vi "TimeOut.vi"(9 "IA State":T2={"our_robots"=[], "enemy_robots"=[], "balls"=[], "geometry"={"field_length"=0, "field_width"=0, "goal_width"=0, "goal_depth"=0, "center_circle_radius"=0, "defense_width"=0, "defense_depth"=0, "free_kick_from_defense_dist"=0, "penalty_spot_from_field_line_dist"=0, "penalty_line_from_spot_dist"=0, "half_moon_depth"=0, "half_moon_width"=0}, "IA Judge"={"stage"="", "command"="", "our_goalie_id"=0.0, "enemy_goalie_id"=0.0, "command enum"=enum."Halt", "Time"=enum."Azul"}, "Received Timestamp"=timestamp(0 s since 1904-01-01), "Events"={"Touch"=FALSE, "id touch"=0.0, "Ball out of \nVision"=FALSE, "Ball inside \nGoalie area"=FALSE, "Robot not responding"=FALSE, "Robots responding status"=[1.0, 1.0, 1.0, 1.0, 1.0, 1.0], "Enemy Ball \nPossession"=FALSE, "Id ini Possession"=0.0, "Ball Possesion"=FALSE, "Id Possesion"=0.0, "Ball at\nour goal side"=FALSE, "Ball at\ntouchline"=FALSE, "Ball at\nenemy goal side"=FALSE}}, 10 "balls":T1[](array[typedef]), 11 "Robot in":T3) -> (3 "Robot out":T3)   [LabVIEW 2018]
uses:
  AI Parameters.ctl
  Core/AI Robot.ctl
  Functions Enum.ctl
  AttackerStates.ctl
  Path Planning/RRT/PathDests.ctl
  Path Planning/RRT/PathDest.ctl
  Core/AI Input.ctl
  Core/AI Ball.ctl
  Core/Field Size.ctl
  Core/AI Judge.ctl
  Command Enum.ctl
  Util/Events/Events.ctl
panel:
  in  "AI Parameters":T12={"GotoKick"={"Dist do cone a frente"=0.0, "attacker farback"=1000.0, "Perto"=300.0, "min dist to kick"=0.0, "kick eps"=110.0, "Time to transition"=0.05}, "Attacker"={"CC chute"=0.09, "CC passe"=0.045, "Kick Force"=200.0, "D ball-robot Kick"=200.0, "D ball-robot Pass"=0.0}, "Defender"={"D max"=1700.0, "Vel p/ robô av"=1000.0, "Kick Force"=100.0, "D atk-def"=300.0, "D farback"=400.0}, "Timeout"={"Field/v in x"=6.0, "Dist Robots"=300, "Dist up in y"=300}, "Pose Striker"={"dist"=200.0, "Numeric"=-4.0, "dist 2"=200.0}, "Dist Stop"=300.0, "Distance when ball out"=200, "D central gap "=150.0, "T pass"=0.0, "Force ++"=0.0, "range kick"=0.0, "Chute alto"=TRUE, "Marcador novo"=TRUE} {"D central gap" format="%#_13g"; "Dist Stop" format="%#_13g"; "Pose Striker"."Numeric" format="%#_13g"; "Defender"."Kick Force" format="%#_13g"; "Defender"."Vel p/ robô av" format="%#_13g"; "Attacker"."D ball-robot Kick" format="%#_13g"; "Attacker"."Kick Force" format="%#_13g"; "Attacker"."CC passe" format="%#_13g"; "Attacker"."CC chute" format="%#_13g"; "GotoKick"."min dist to kick" format="%#_13g"; "GotoKick"."Perto" format="%#_13g"; "GotoKick"."attacker farback" format="%#_13g"; "GotoKick"."Dist do cone a frente" format="%#_13g"}
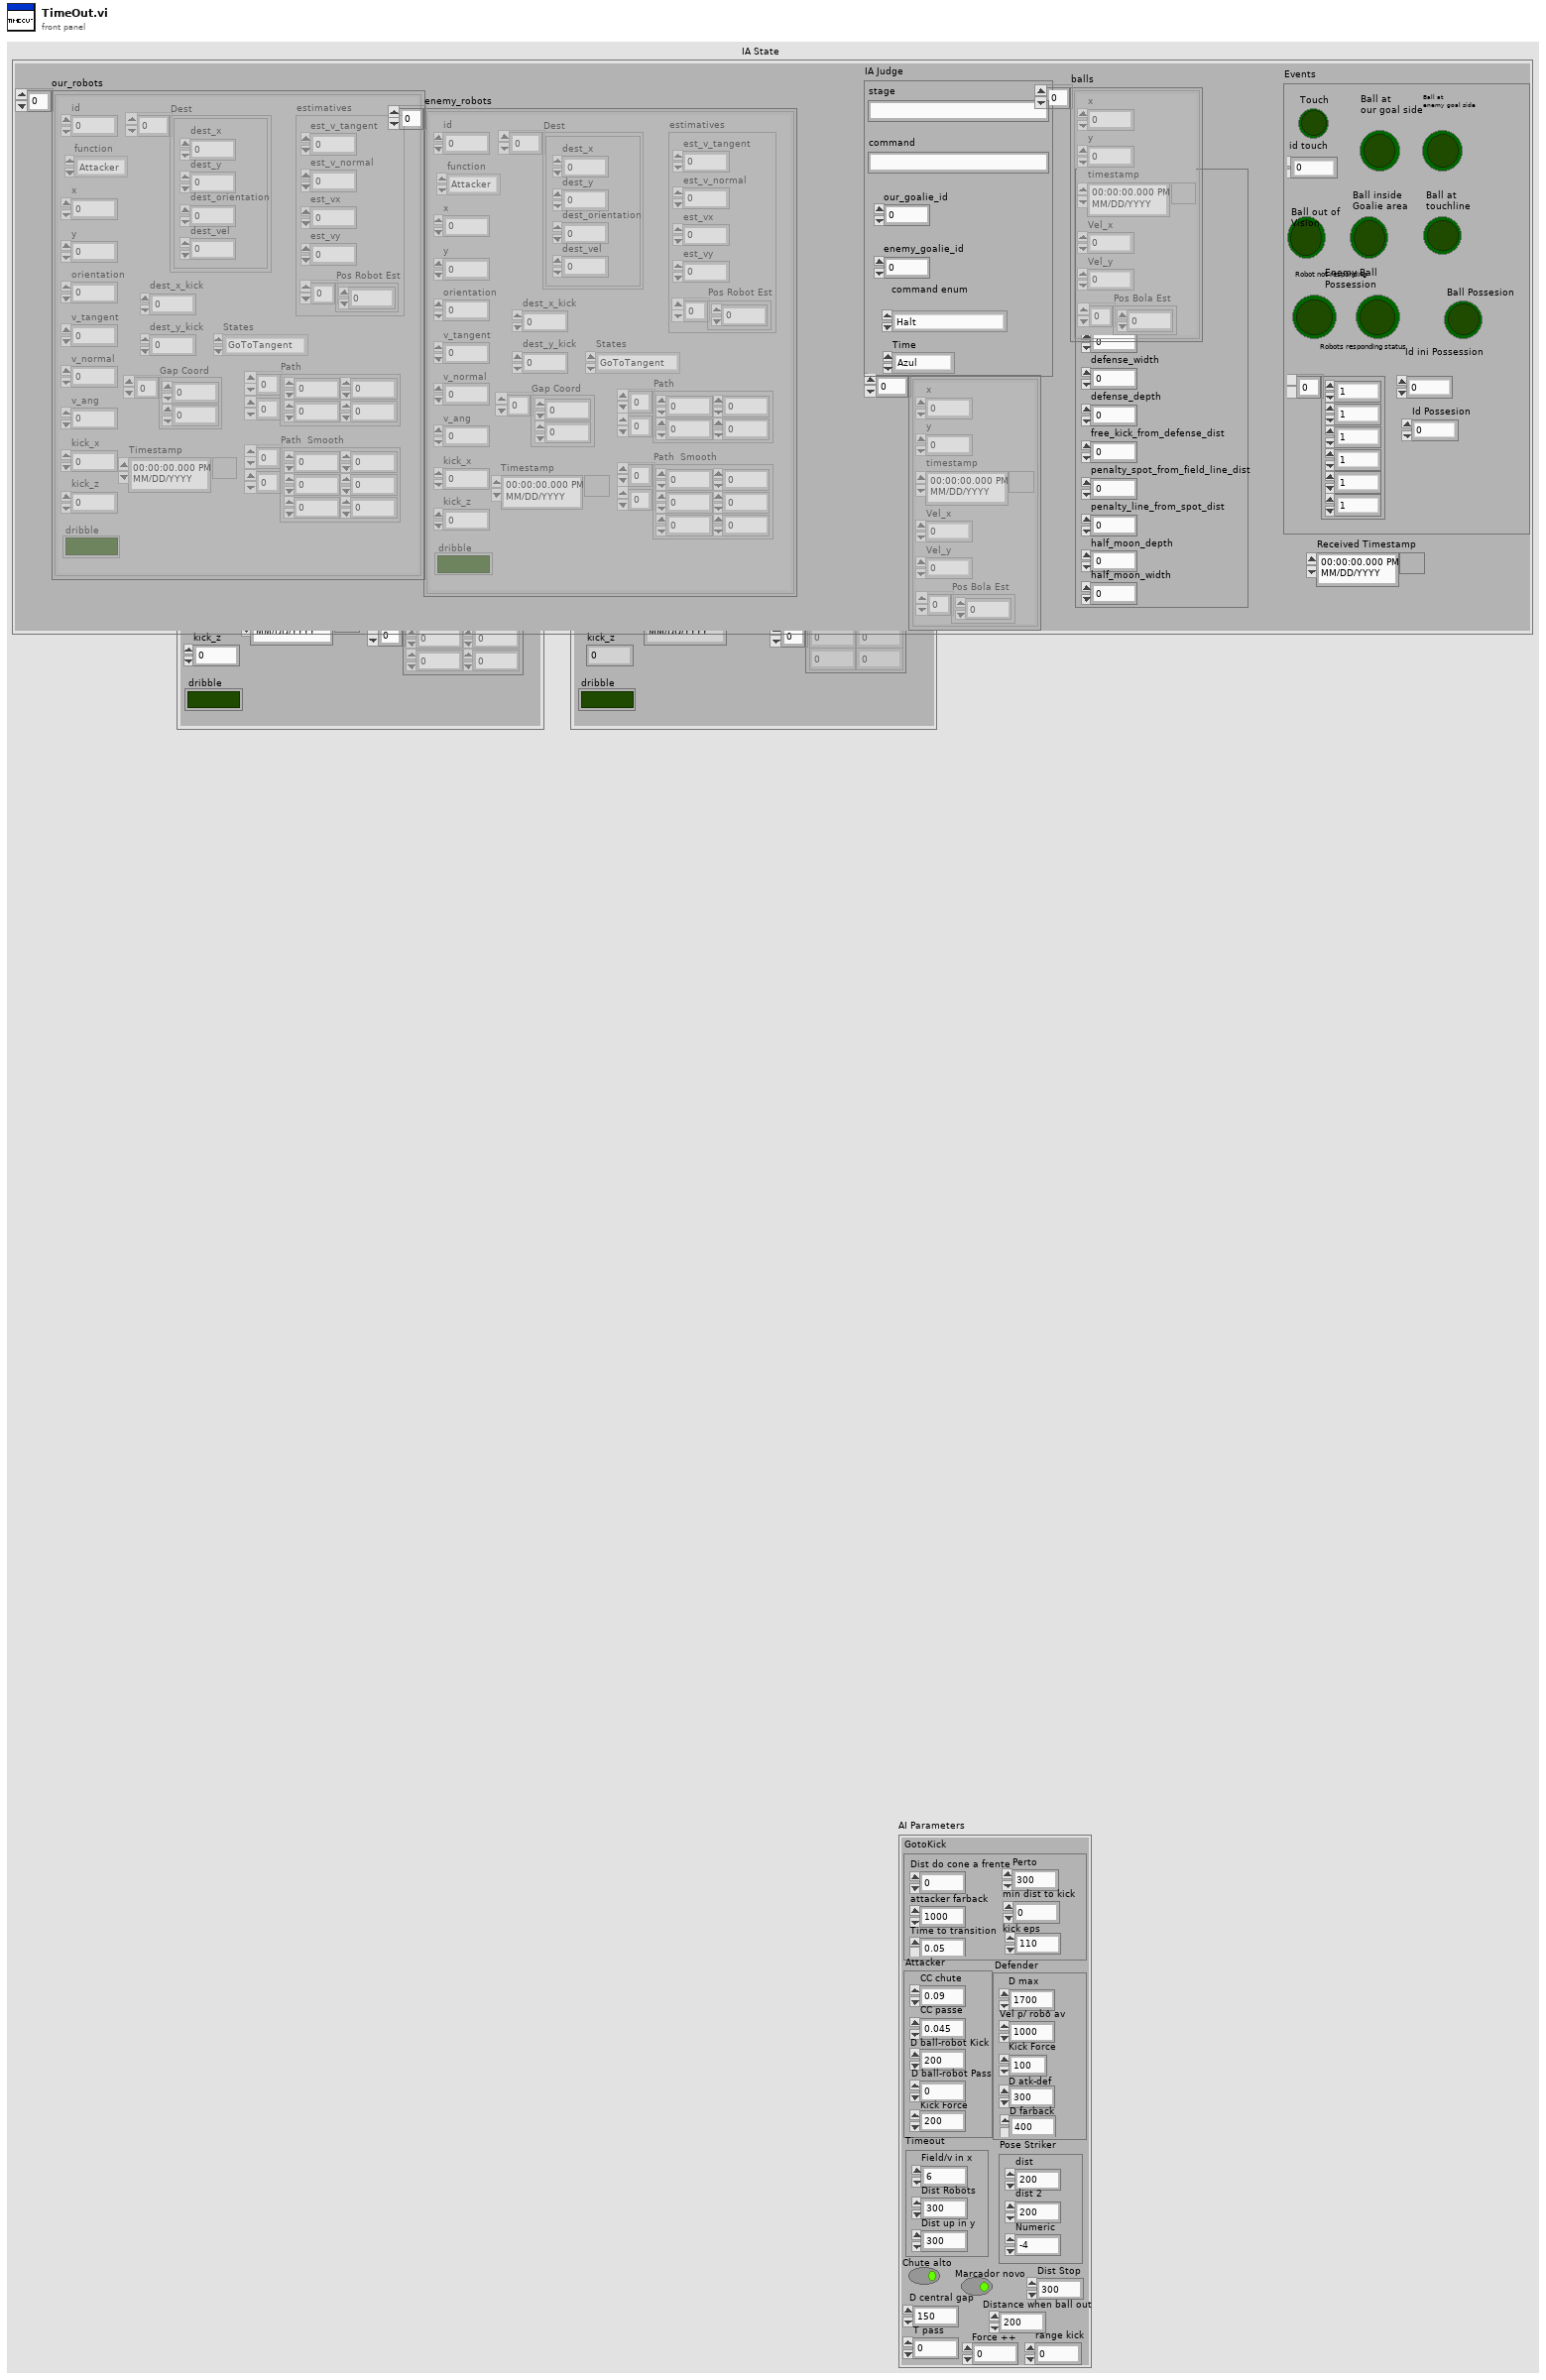
[diagram p1: front panel]
types:
  T1 = typedef "AI Ball.ctl" = cluster{"x":dbl, "y":dbl, "timestamp":timestamp, "Vel_x":dbl, "Vel_y":dbl, "Pos Bola Est":dbl[]}
  T2 = typedef "AI Input.ctl" = cluster{"our_robots":T3[], "enemy_robots":T3[], "balls":T1[], "geometry":T8, "IA Judge":T9, "Received Timestamp":timestamp, "Events":T11}
  T3 = typedef "AI Robot.ctl" = cluster{"id":u32, "function":T4, "x":dbl, "y":dbl, "orientation":dbl, "v_tangent":dbl, "v_normal":dbl, "v_ang":dbl, "kick_x":dbl, "kick_z":dbl, "dribble":bool, "Timestamp":timestamp, "estimatives":cluster{"est_v_tangent":dbl, "est_v_normal":dbl, "est_vx":dbl, "est_vy":dbl, "Pos Robot Est":dbl[]}, "dest_x_kick":dbl, "dest_y_kick":dbl, "Gap Coord":dbl[], "States":T5, "Path ":dbl[][], "Path  Smooth":dbl[][], "Dest":T6}
  T4 = typedef "Functions Enum.ctl" = enum16{"Attacker", "Goalie", "Defender", "Striker", "Goto 0", "Dummy", "Kicker", "ZigZag"}
  T5 = typedef "AttackerStates.ctl" = enum16{"Pass", "GoToTangent", "BallGetting", "GoToKick", "Rotate anti-clockwise", "Rotate Clockwise", ""}
  T6 = typedef "PathDests.ctl" = T7[]
  T7 = typedef "PathDest.ctl" = cluster{"dest_x":dbl, "dest_y":dbl, "dest_orientation":dbl, "dest_vel":dbl}
  T8 = typedef "Field Size.ctl" = cluster{"field_length":u32, "field_width":u32, "goal_width":u32, "goal_depth":u32, "center_circle_radius":u32, "defense_width":u32, "defense_depth":u32, "free_kick_from_defense_dist":u32, "penalty_spot_from_field_line_dist":u32, "penalty_line_from_spot_dist":u32, "half_moon_depth":u32, "half_moon_width":u32}
  T9 = typedef "AI Judge.ctl" = cluster{"stage":string, "command":string, "our_goalie_id":dbl, "enemy_goalie_id":dbl, "command enum":T10, "Time":enum16{"Azul", "Amarelo"}}
  T10 = typedef "Command Enum.ctl" = enum16{"Halt", "Stop", "Force Start", "PKA Normal Start", "Prepare Kickoff Ally", "PKE Normal Start", "Prepare Kickoff Enemy", "Prepare Penalty Ally", "PPA Normal Start", "Prepare Penalty Enemy", "PPE Normal Start", "Ball Placement Enemy Up", "Ball Placement Enemy Down", "Ball Placement Ally Up", "Ball Placement Ally Mid", "Ball Placement Ally Down", "Indirect Free Enemy", "Indirect Free Ally", "Timeout Enemy", "Timeout Ally", "Goal Enemy", "Goal Ally", "Normal Half Time", "Extra Time Break", "Extra Half Time", "None", "Post Game"}
  T11 = typedef "Events.ctl" = cluster{"Touch":bool, "id touch":dbl, "Ball out of \nVision":bool, "Ball inside \nGoalie area":bool, "Robot not responding":bool, "Robots responding status":dbl[], "Enemy Ball \nPossession":bool, "Id ini Possession":dbl, "Ball Possesion":bool, "Id Possesion":dbl, "Ball at\nour goal side":bool, "Ball at\ntouchline":bool, "Ball at\nenemy goal side":bool}
  T12 = typedef "AI Parameters.ctl" = cluster{"GotoKick":cluster{"Dist do cone a frente":dbl, "attacker farback":dbl, "Perto":dbl, "min dist to kick":dbl, "kick eps":dbl, "Time to transition":dbl}, "Attacker":cluster{"CC chute":dbl, "CC passe":dbl, "Kick Force":dbl, "D ball-robot Kick":dbl, "D ball-robot Pass":dbl}, "Defender":cluster{"D max":dbl, "Vel p/ robô av":dbl, "Kick Force":dbl, "D atk-def":dbl, "D farback":dbl}, "Timeout":cluster{"Field/v in x":dbl, "Dist Robots":u32, "Dist up in y":u32}, "Pose Striker":cluster{"dist":dbl, "Numeric":dbl, "dist 2":dbl}, "Dist Stop":dbl, "Distance when ball out":i32, "D central gap ":dbl, "T pass":dbl, "Force ++":dbl, "range kick":dbl, "Chute alto":bool, "Marcador novo":bool}
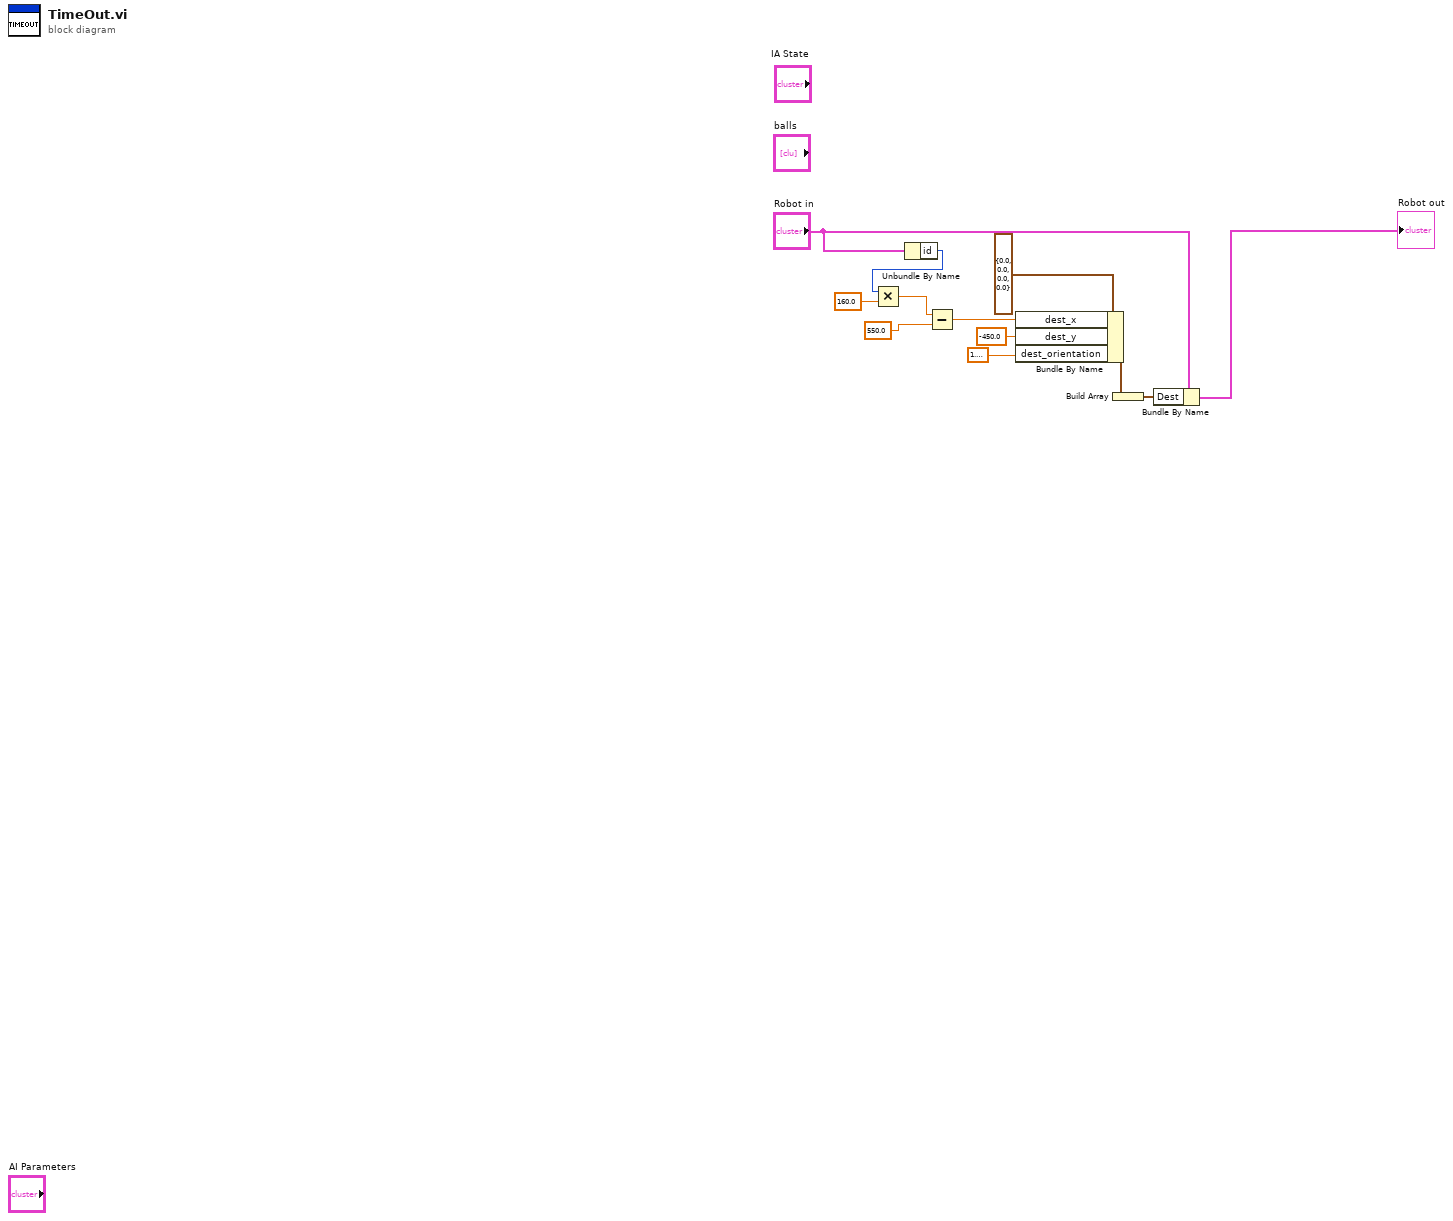
[diagram p0: block diagram]
diagram:
  n1 = Unbundle By Name("Robot in") -> ("id"=w5:u32)
  n2 = Multiply(x=w5, y=160.0) -> (x*y=w4:dbl)
  n3 = Subtract(x=w4, y=550.0) -> (x-y=w1:dbl)
  n4 = Bundle By Name(cluster=T7 {"dest_x"=0.0, "dest_y"=0.0, "dest_orientation"=0.0, "dest_vel"=0.0} ("element"), "dest_x"=w1, "dest_y"=-450.0, "dest_orientation"=1.5707963267948966) -> (w10:T7)
  n5 = Build Array(w10) -> (w11:T7[])
  n6 = Bundle By Name(cluster="Robot in", "Dest"=w11) -> (→"Robot out":T3)
